vi "test CopyEqualSize.vi"(8 "error in (no error)":errorcluster, 11 "TestCase in":refnum<class "Data Manipulation Tests.lvclass">) -> (0 "error out":errorcluster, 3 "TestCase out":refnum<class "Data Manipulation Tests.lvclass">)   [LabVIEW 2017, in "Pointer Tests.lvlib" / "Data Manipulation Tests.lvclass"]
uses:
  Data Manipulation Tests.lvclass
  Source/Classes/Pointer/Public/New/New (4B).vi
  Source/Classes/Pointer/Public/Write/Write (1D I32).vi
  <vilib>/addons/_JKI Toolkits/VI Tester/TestCase.llb/TestCase.lvclass
  Source/Classes/Pointer/Pointer.lvclass
  C:/Program Files (x86)/National Instruments/LabVIEW 2017/vi.lib/addons/_JKI Toolkits/VI Tester/TestCase.llb/TestCase.lvclass
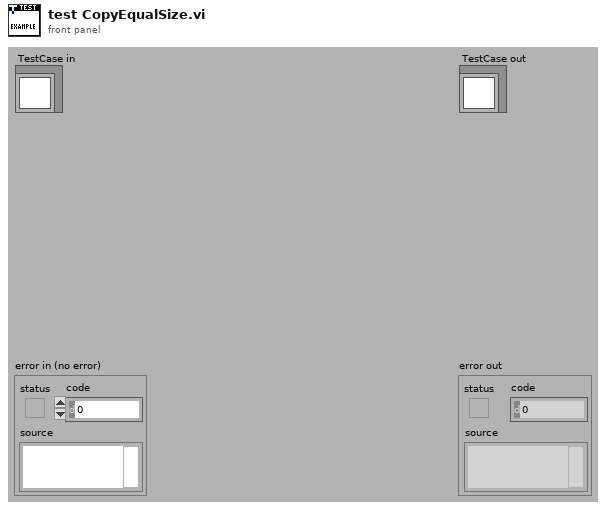
[diagram p1: front panel]
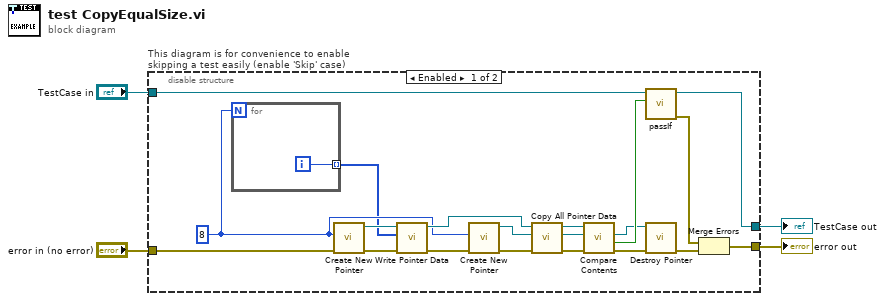
[diagram p0: block diagram]
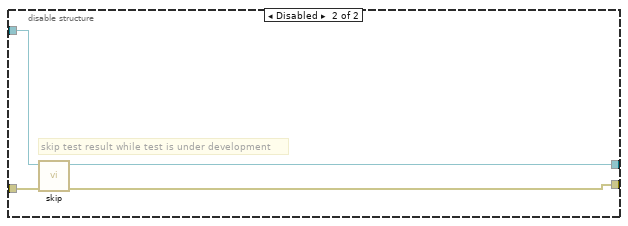
[diagram p2: hidden frame]
diagram:
  n1 = disable-structure "This diagram is for convenience to enable skipping a test easily (enable 'Skip' case)" shown="Enabled" {
    disable-tunnel: "TestCase in" -> [w16 w29]
    disable-tunnel: [w15 w27] -> w1
    disable-tunnel: [w9 w28] -> w3
    disable-tunnel: "error in (no error)" -> [w13 w26]
    frame Enabled {
      w22 = u64 8 ("count (1)")
      n2 = for {
        N: w22 -> [_]
        tunnel: [w25] -> w21 mode=indexing
        i -> [w25]
      }
      n3 = call-poly "Create New Pointer.vi"("error in (no error)"=w13, "count (1)"=w22) -> ("error out"=w12:errorcluster, "Pointer"=w24:refnum<class "Pointer.lvclass">)  [unwired: 8 in]
      n4 = call-poly "Write Pointer Data.vi"("error in (no error)"=w12, "buffer in"=w21, "Pointer in"=w24) -> ("error out"=w11:errorcluster, "Pointer out"=w23:refnum<class "Pointer.lvclass">)  [unwired: 5 in, 2 out]
      n5 = call-poly "Create New Pointer.vi"("error in (no error)"=w11, "count (1)"=w22) -> ("error out"=w10:errorcluster, "Pointer"=w20:refnum<class "Pointer.lvclass">)  [unwired: 8 in]
      n6 = call "Copy All Pointer Data.vi"("error in (no error)"=w10, "dst Pointer in"=w20, "src Pointer in"=w23) -> ("error out"=w7:errorcluster, "dst Pointer out"=w18:refnum<class "Pointer.lvclass">, "src Pointer out"=w19:refnum<class "Pointer.lvclass">)  [unwired: 6 in]
      n7 = call "Compare Contents.vi"("error in (no error)"=w7, "Pointer b in"=w18, "Pointer a in"=w19) -> ("error out"=w8:errorcluster, "equal contents?"=w14:bool, "Pointer b out"=w5:refnum<class "Pointer.lvclass">)  [unwired: 5 in, 1 out]
      n8 = call-dynamic "passIf.vi"("pass"=w14, "TestCase in"=w16) -> ("error out"=w17:errorcluster, "TestCase out"=w15:refnum<class "Data Manipulation Tests.lvclass">)  [unwired: 8 in]
      n9 = call "Destroy Pointer.vi"("error in (no error)"=w8, "Pointer in"=w5) -> ("error out"=w6:errorcluster)  [unwired: 8 in, 1 out]
      n10 = Merge Errors(w17, w6) -> (w9:errorcluster)
    }
    frame Disabled {
      # "skip test result while test is under development"
      n11 = call <vilib>:"skip.vi"("error in (no error)"=w26, "TestCase in"=w29) -> ("error out"=w28:errorcluster, "TestCase out"=w27:refnum<class "Data Manipulation Tests.lvclass">)  [unwired: 8 in]
    }
  }
  "error out" <- w3
  "TestCase out" <- w1
